vi "Fsk.vi"() -> ()   [LabVIEW 2013]
panel:
  out "Fsk":dbl
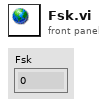
[diagram p1: front panel]
diagram:
